vi "Get Variables.vi"(8 "error in (no error)":errorcluster, 11 "Message Popup in":refnum<class "ControllerData.lvclass">) -> (0 "error out":errorcluster, 2 "Variables":variant, 3 "Message Popup out":refnum<class "ControllerData.lvclass">)   [LabVIEW 2019, in "ControllerData.lvclass"]
uses:
  ControllerData.lvclass
  ControllerData.lvclass/ControllerData.ctl
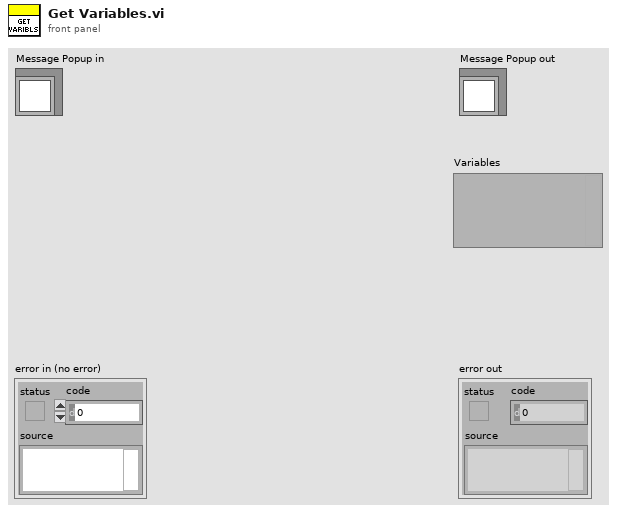
[diagram p1: front panel]
types:
  T1 = typedef "ControllerData.lvclass/Variables.ctl" = cluster{"PreviousValues":i32}
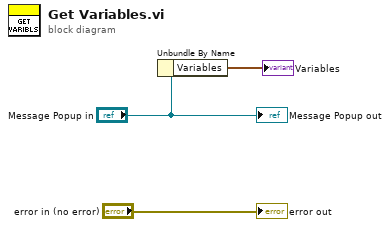
[diagram p0: block diagram]
diagram:
  n1 = Unbundle By Name("Message Popup in") -> ("Variables"=→"Variables":T1)
  "error out" <- "error in (no error)"
  "Message Popup out" <- "Message Popup in"
